vi "UI_checkChar.vi"(9 "Buying Vowel?":bool, 11 "Char":i16) -> (2 "Char OK?":bool)   [LabVIEW 2020]
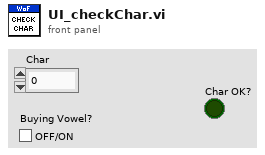
[diagram p1: front panel]
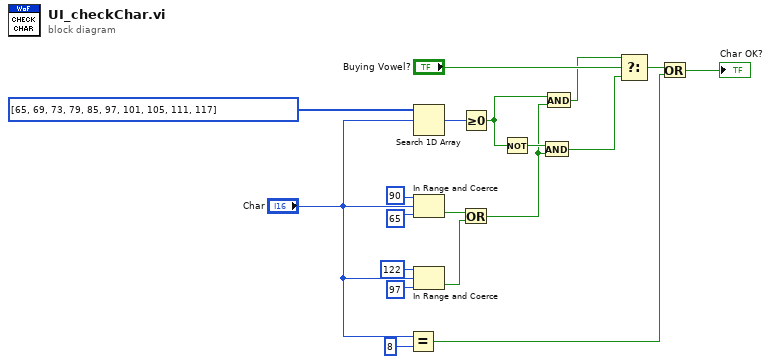
[diagram p0: block diagram]
diagram:
  n1 = Equal?(x="Char", y=i16 8) -> (x = y?=w1:bool)
  n2 = Search 1D Array(1D array=i16[] [65, 69, 73, 79, 85, 97, 101, 105, 111, 117], element="Char") -> (index of element=w12:i32)  [unwired: 1 in]
  n3 = In Range and Coerce(upper limit=i16 90, x="Char", lower limit=i16 65) -> (In Range?=w14:bool)  [unwired: 1 out]
  n4 = In Range and Coerce(upper limit=i16 122, x="Char", lower limit=i16 97) -> (In Range?=w13:bool)  [unwired: 1 out]
  n5 = Greater Or Equal To 0?(x=w12) -> (x >= 0?=w7:bool)
  n6 = Or(x=w14, y=w13) -> (x .or. y?=w8:bool)
  n7 = Not(x=w7) -> (.not. x?=w10:bool)
  n8 = And(x=w10, y=w8) -> (x .and. y?=w9:bool)
  n9 = And(x=w7, y=w8) -> (x .and. y?=w6:bool)
  n10 = Select(t=w6, s="Buying Vowel?", f=w9) -> (s? t:f=w3:bool)
  n11 = Or(x=w3, y=w1) -> (x .or. y?=→"Char OK?":bool)
